vi "BRig_dataCurrent_L_ENL2_T_start_l1.vi"() -> (2 "output_L_ENL2_T_start_l1":i32)   [LabVIEW 2014]
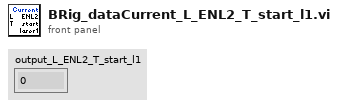
[diagram p1: front panel]
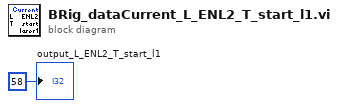
[diagram p0: block diagram]
diagram:
  "output_L_ENL2_T_start_l1" <- 58 ("output_iBlock")
